vi "Read Exporter.vi"(9 "Selection":string, 11 "UIManager in":refnum<class "UIManager.lvclass">) -> (0 "error out":errorcluster, 1 "Parameters":string, 2 "IExporter.lvclass":refnum<class "IExporter.lvclass">, 3 "UIManager out":refnum<class "UIManager.lvclass">, 4 "found?":bool)   [LabVIEW 2020, in "UserInterface.lvlib" / "UIManager.lvclass"]
uses:
  UIManager.lvclass
  ExtensionInterfaces/IExporter/IExporter.lvclass
  UIManager.lvclass/UIManager.ctl
  c4c521ad-ffdb-46af-ac16-6752d92c70ba.vi
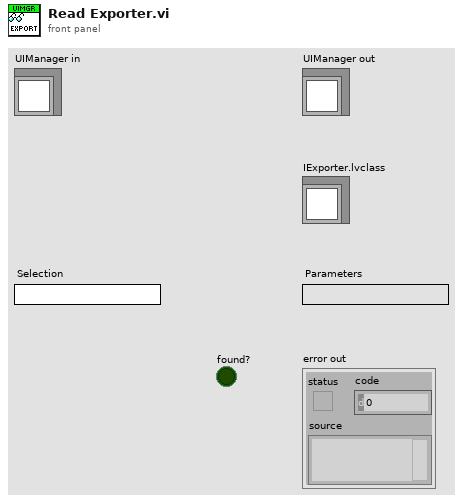
[diagram p1: front panel]
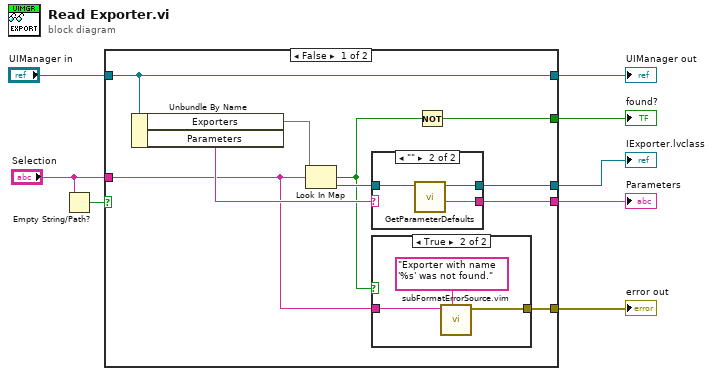
[diagram p0: block diagram]
diagram:
  n1 = Empty String/Path?(string/path="Selection") -> (empty?=w2:bool)
  n2 = case shown="False" w2 {
    tunnel: "UIManager in" -> [w9 w27]
    tunnel: [w17 _] -> w7
    tunnel: [w14 _] -> w6
    tunnel: [w13 _] -> w5
    tunnel: "Selection" -> [w11 _]
    tunnel: [w10 _] -> w4
    tunnel: [w9 w27] -> w1
    frame False {
      n3 = Unbundle By Name(w9) -> ("Exporters"=w18:map{string, refnum<class "IExporter.lvclass">}, "Parameters"=w16:string)
      n4 = Look In Map(map=w18, key=w11) -> (key not found?=w12:bool, value=w15:refnum<class "IExporter.lvclass">)  [unwired: 1 in]
      n5 = case shown="\"\"" w16 {
        selector: w16 -> [w23 _]
        tunnel: [w23 w25] -> w13
        tunnel: w15 -> [w22 w26]
        tunnel: [w22 w24] -> w14
        frame Default {
        }
        frame "" {
          n6 = call-dynamic "GetParameterDefaults.vi"("IExporter in"=w26) -> ("Parameter defaults"=w25:string, "IExporter out"=w24:refnum<class "IExporter.lvclass">)  [unwired: 8 in, 1 out]
        }
      }
      n7 = case shown="True" w12 {
        tunnel: [_ w19] -> w10
        tunnel: w11 -> [_ w20]
        frame False {
        }
        frame True {
          n8 = call "subFormatErrorSource.vim"("format string"="Exporter with name '%s' was not found.", "Parameter cluster"=w20) -> ("Error out"=w19:errorcluster)  [unwired: 9 in]
        }
      }
      n9 = Not(x=w12) -> (.not. x?=w17:bool)
    }
    frame True {
    }
  }
  "UIManager out" <- w1
  "IExporter.lvclass" <- w6
  "found?" <- w7
  "Parameters" <- w5
  "error out" <- w4
